vi "write16bitTiff_withtext.vi"(2 "16-bit pixmap x, y":u16[][](array[numeric]), 3 "Text":string, 4 "file path":path) -> (0 "error out":errorcluster)   [LabVIEW 2011]
uses:
  TiffModules/AddTiffPage_U16_text.vi
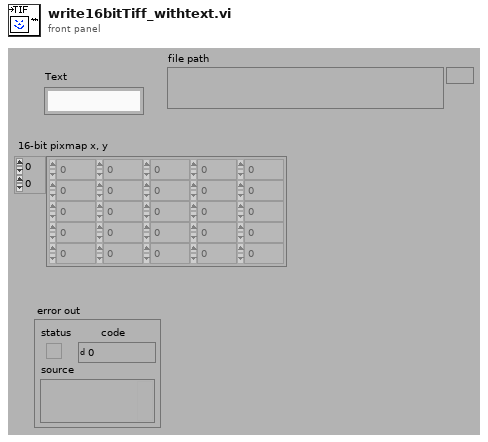
[diagram p1: front panel]
types:
  T1 = cluster{"Tiff refnum":refnum<file>, "BigTiff,Endian":u16}
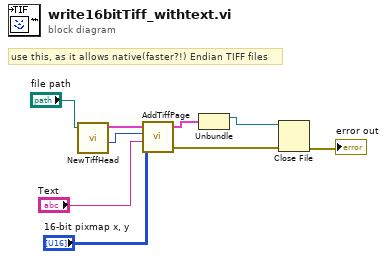
[diagram p0: block diagram]
diagram:
  # "use this, as it allows native(faster?!) Endian TIFF files"
  n1 = call "NewTiffHead.vi"("file path"="file path") -> ("TIFF file"=w7:T1, "Place for first IFD (8,eof-position)"=w6:u64)  [unwired: 2 in, 2 out]
  n2 = call-poly "AddTiffPage.vi"("TIFF file"=w7, "After last DIROffset"=w6, "Text"="Text", "16-bit pixmap x, y"="16-bit pixmap x, y") -> ("TIFF file"=w3:T1, "error out"=w1:errorcluster)  [unwired: 2 out]
  n3 = Unbundle(w3) -> ("Tiff refnum"=w2:refnum<file>)  [unwired: 1 out]
  n4 = Close File(refnum=w2, error in=w1) -> (error out=→"error out":errorcluster)  [unwired: 1 out]
